vi "simulator_commands_no_msgpack.vi"() -> ()   [LabVIEW 2018]
panel:
  out "message_length":u32
  out "String":string
  out "bytes written":i32
  out "data out":string
  in  "Simulator Configuration":path=path "C:/Users/celit/Documents/GitHub/client/configurations/simulator.json"
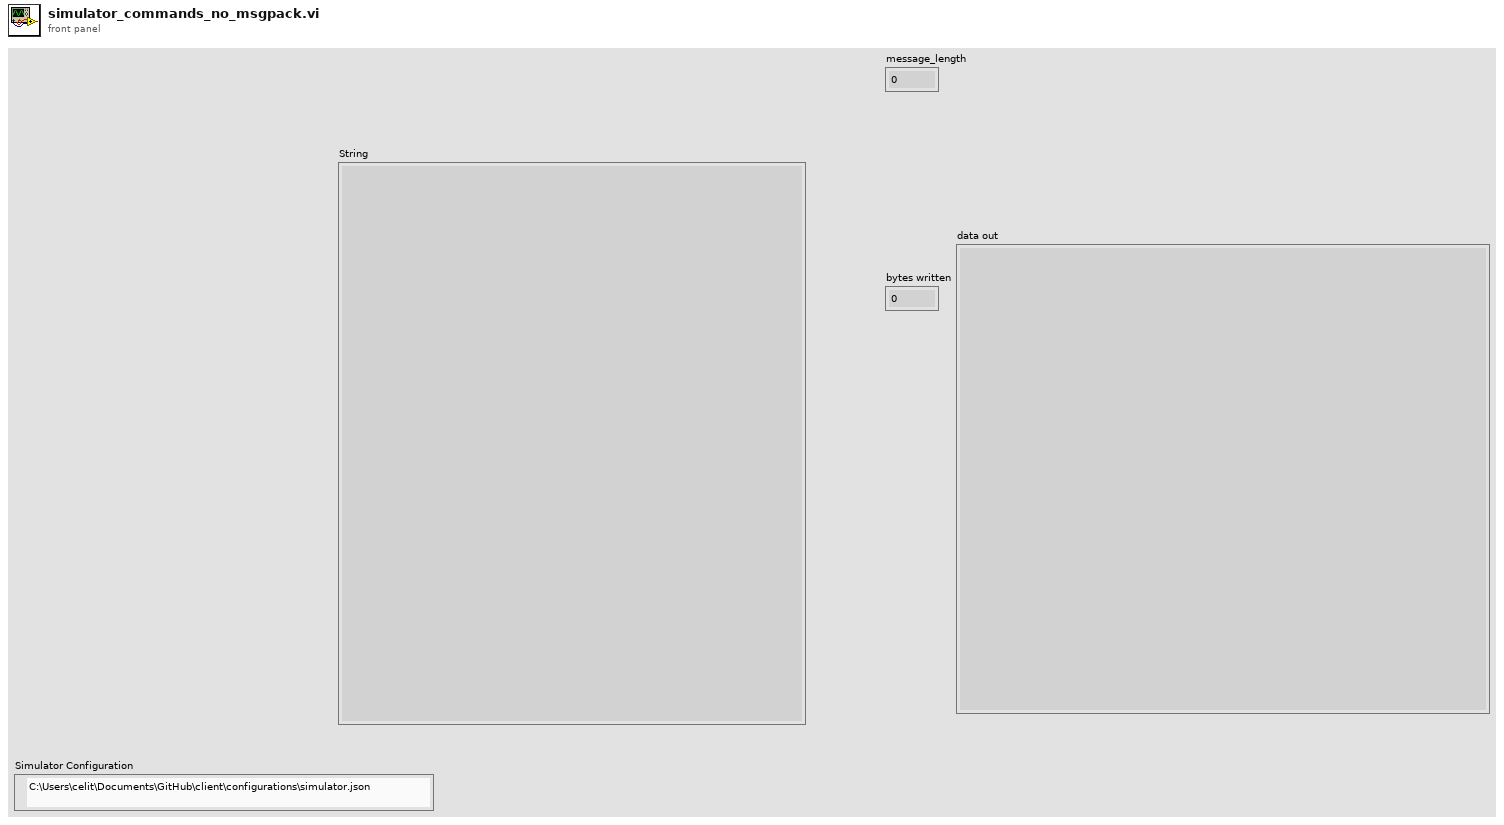
[diagram p1: front panel]
types:
  T1 = cluster{"class":string, "status":string, "messages":string, "data":string}
  T2 = cluster{"id":string, "server_ip":string, "server_port":i32, "client_ip":string}
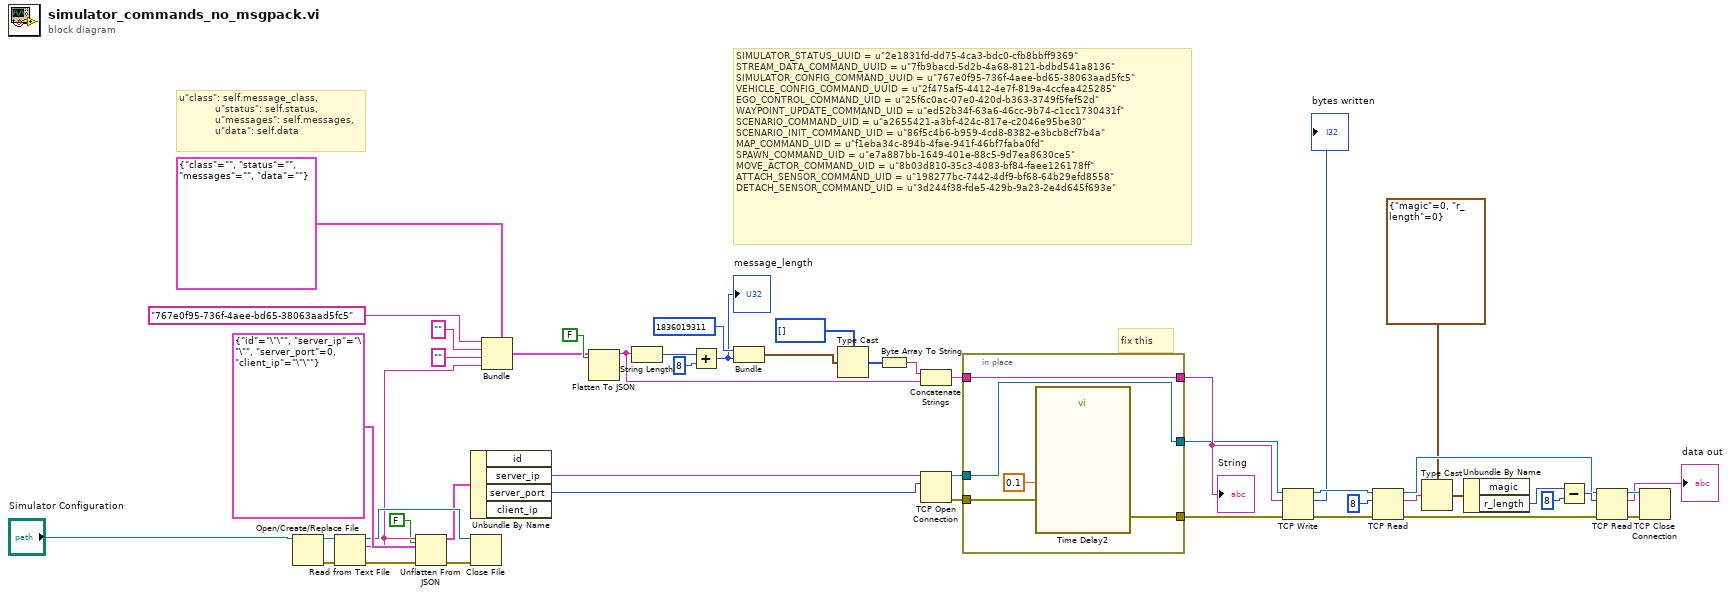
[diagram p0: block diagram]
diagram:
  # "fix this"
  # "u\"class\": self.message_class,\n            u\"status\": self.status,\n            u\"messages\": self.messages,\n            u\"data\": self.data"
  # "SIMULATOR_STATUS_UUID = u\"2e1831fd-dd75-4ca3-bdc0-cfb8bbff9369\"\nSTREAM_DATA_COMMAND_UUID = u\"7fb9bacd-5d2b-4a68-8121-bdbd541a8136\"\nSIMULATOR_CONFIG_COMMAND_UUID = u\"767e0f95-736f-4aee-bd65-38063aad5fc5\"\nVEHICLE_CONFIG_COMMAND_UUID = u\"2f475af5-4412-4e7f-819a-4ccfea425285\"\nEGO_CONTROL_COMMAND_UID = u\"25f6c0ac-07e0-420d-b363-3749f5fef52d\"\nWAYPOINT_UPDATE_COMMAND_UID = u\"ed52b34f-63a6-46cc-9b74-c1cc1730431f\"\nSCENARIO_COMMAND_UID = u\"a2655421-a3bf-424c-817e-c2046e95be30\"\nSCENARIO_INIT_COMMAND_UID = u\"86f5c4b6-b959-4cd8-8382-e3bcb8cf7b4a\"\nMAP_COMMAND_UID = u\"f1eba34c-894b-4fae-941f-46bf7faba0fd\"\nSPAWN_COMMAND_UID = u\"e7a887bb-1649-401e-88c5-9d7ea8630ce5\"\nMOVE_ACTOR_COMMAND_UID = u\"8b03d810-35c3-4083-bf84-faee126178ff\"\nATTACH_SENSOR_COMMAND_UID = u\"198277bc-7442-4df9-bf68-64b29efd8558\"\nDETACH_SENSOR_COMMAND_UID = u\"3d244f38-fde5-429b-9a23-2e4d645f693e\""
  n1 = Open/Create/Replace File(file path (use dialog)="Simulator Configuration") -> (refnum out=w41:refnum<file>, error out=w40:errorcluster)  [unwired: 5 in, 1 out]
  n2 = Read from Text File(file (use dialog)=w41, error in=w40) -> (refnum out=w37:refnum<file>, text=w33:string, error out=w38:errorcluster)  [unwired: 2 in, 1 out]
  n3 = Unflatten From JSON(enable LabVIEW extensions? (T)=FALSE, JSON string=w33, type and defaults=T2 {"id"="\"\"", "server_ip"="\"\"", "server_port"=0, "client_ip"="\"\""}, error in (no error)=w38) -> (value=w36:T2, error out=w39:errorcluster)  [unwired: 3 in]
  n4 = Unbundle By Name(w36) -> ("server_ip"=w30:string, "server_port"=w29:i32)  [unwired: 2 out]
  n5 = Close File(refnum=w37, error in=w39) -> ()  [unwired: 2 out]
  n6 = Bundle(cluster=T1 {"class"="", "status"="", "messages"="", "data"=""}, "class"="767e0f95-736f-4aee-bd65-38063aad5fc5", "status"="", "messages"="", "data"=w33) -> (w34:T1)
  n7 = Flatten To JSON(enable LabVIEW extensions? (T)=FALSE, anything=w34) -> (JSON string=w2:string)  [unwired: 1 in, 1 out]
  n8 = String Length(string=w2) -> (length=w1:i32)
  n9 = Add(x=w1, y=u32 8) -> (x+y=w22:u32)
  "message_length" <- w22
  n10 = Bundle(u32 1836019311, w22) -> (w28:cluster{u32, u32})  [unwired: 1 in]
  n11 = Type Cast(type=u8[] [], x=w28) -> (*(type *) &x=w26:u8[])
  n12 = Byte Array To String(unsigned byte array=w26) -> (string=w20:string)
  n13 = Concatenate Strings(w20, w2) -> (w18:string)
  n14 = TCP Open Connection(address=w30, remote port or service name=w29) -> (connection ID=w15:refnum<k5>, error out=w19:errorcluster)  [unwired: 3 in]
  n15 = in-place {
    in-place-border: [w53] -> w14
    in-place-border: w19 -> [w52]
    in-place-border: w18 -> [w51]
    in-place-border: [w51] -> w17
    in-place-border: [w50] -> w16
    in-place-border: w15 -> [w50]
    n16 = call "Time Delay2"("error in (no error)"=w52, "Delay Time (s)"=0.1) -> ("error out"=w53:errorcluster)  [unwired: 9 in]
  }
  "String" <- w17
  n17 = TCP Write(connection ID=w16, data in=w17, error in (no error)=w14) -> (connection ID out=w42:refnum<k5>, bytes written=→"bytes written":i32, error out=w45:errorcluster)  [unwired: 1 in]
  n18 = TCP Read(connection ID=w42, bytes to read=8, error in (no error)=w45) -> (connection ID out=w8:refnum<k5>, data out=w13:string, error out=w9:errorcluster)  [unwired: 2 in]
  n19 = Type Cast(type=cluster{"magic":u32, "r_length":u32} {"magic"=0, "r_length"=0}, x=w13) -> (*(type *) &x=w12:cluster{"magic":u32, "r_length":u32})
  n20 = Unbundle By Name(w12) -> ("r_length"=w10:u32)  [unwired: 1 out]
  n21 = Subtract(x=w10, y=u32 8) -> (x-y=w11:u32)
  n22 = TCP Read(connection ID=w8, bytes to read=w11, error in (no error)=w9) -> (connection ID out=w43:refnum<k5>, data out=→"data out":string, error out=w44:errorcluster)  [unwired: 2 in]
  n23 = TCP Close Connection(connection ID=w43, error in (no error)=w44) -> ()  [unwired: 1 in, 2 out]
